vi "Follower16_Final.vi"() -> ()   [LabVIEW 2016]
uses:
  <vilib>/NXT/Block Support/NXT_InputPort.ctl
  <vilib>/NXT/Block Support/NXT_TimerIndex.ctl
  <vilib>/NXT/Block Support/NXT_OutputPort.ctl
  <vilib>/NXT/Dual Mode Library/Sensors/EV3_Gyro_Reset.vi
  <vilib>/NXT/Dual Mode Library/Sensors/EV3_Gyro_Angle.vi
  <vilib>/NXT/Dual Mode Library/Sensors/EV3_Gyro_Rate.vi
  <vilib>/NXT/Dual Mode Library/Sensors/Reset_Timer.vi
  <vilib>/NXT/Dual Mode Library/Sensors/EV3_Color_Reflect.vi
  <vilib>/NXT/Dual Mode Library/Sensors/Read_Timer.vi
  <vilib>/NXT/Dual Mode Library/Sensors/EV3_Ultrasonic_CM.vi
  <vilib>/NXT/Dual Mode Library/Display/drawText_Right.vi
  <vilib>/NXT/Dual Mode Library/prims/inRangeAndCoerce/inRangeAndCoerce_float.vi
  <vilib>/NXT/NXTIO Xnodes/NXTIONodeSubVIs/NXTMoveMotors.vi
  <vilib>/NXT/Dual Mode Library/Display/drawNumber.vi
  <vilib>/NXT/Dual Mode Library/Display/drawNumber_float.vi
  <vilib>/NXT/Dual Mode Library/Motors/Rotation.vi
  <vilib>/NXT/Dual Mode Library/Motors/ResetMotor.vi
  <vilib>/NXT/Dual Mode Library/Sensors/Touch_Pressed.vi
  <vilib>/NXT/Dual Mode Library/Sound/PlayC.vi
  <vilib>/NXT/Dual Mode Library/Display/drawText.vi
  <vilib>/NXT/NXTIO Xnodes/NXTIONodeSubVIs/NXTStopMotors.vi
  <vilib>/NXT/Subs/LVHSConnector.ctl
  <vilib>/NXT/NXTIO Xnodes/AddressXNode/NXTIOAddress.xnode
  <vilib>/NXT/NXTIO Xnodes/NXTIOXNode/NXTIO.xnode
  <vilib>/NXT/LegoClasses/BrickReference/BrickReference.lvclass
panel:
  out "Value (msec)":u32
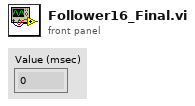
[diagram p1: front panel]
types:
  T1 = typedef "NXT_InputPort.ctl" = u32
  T2 = typedef "LVHSConnector.ctl" = refnum<class "BrickReference.lvclass">
  T3 = typedef "NXT_TimerIndex.ctl" = u8
  T4 = typedef "NXT_OutputPort.ctl" = u8
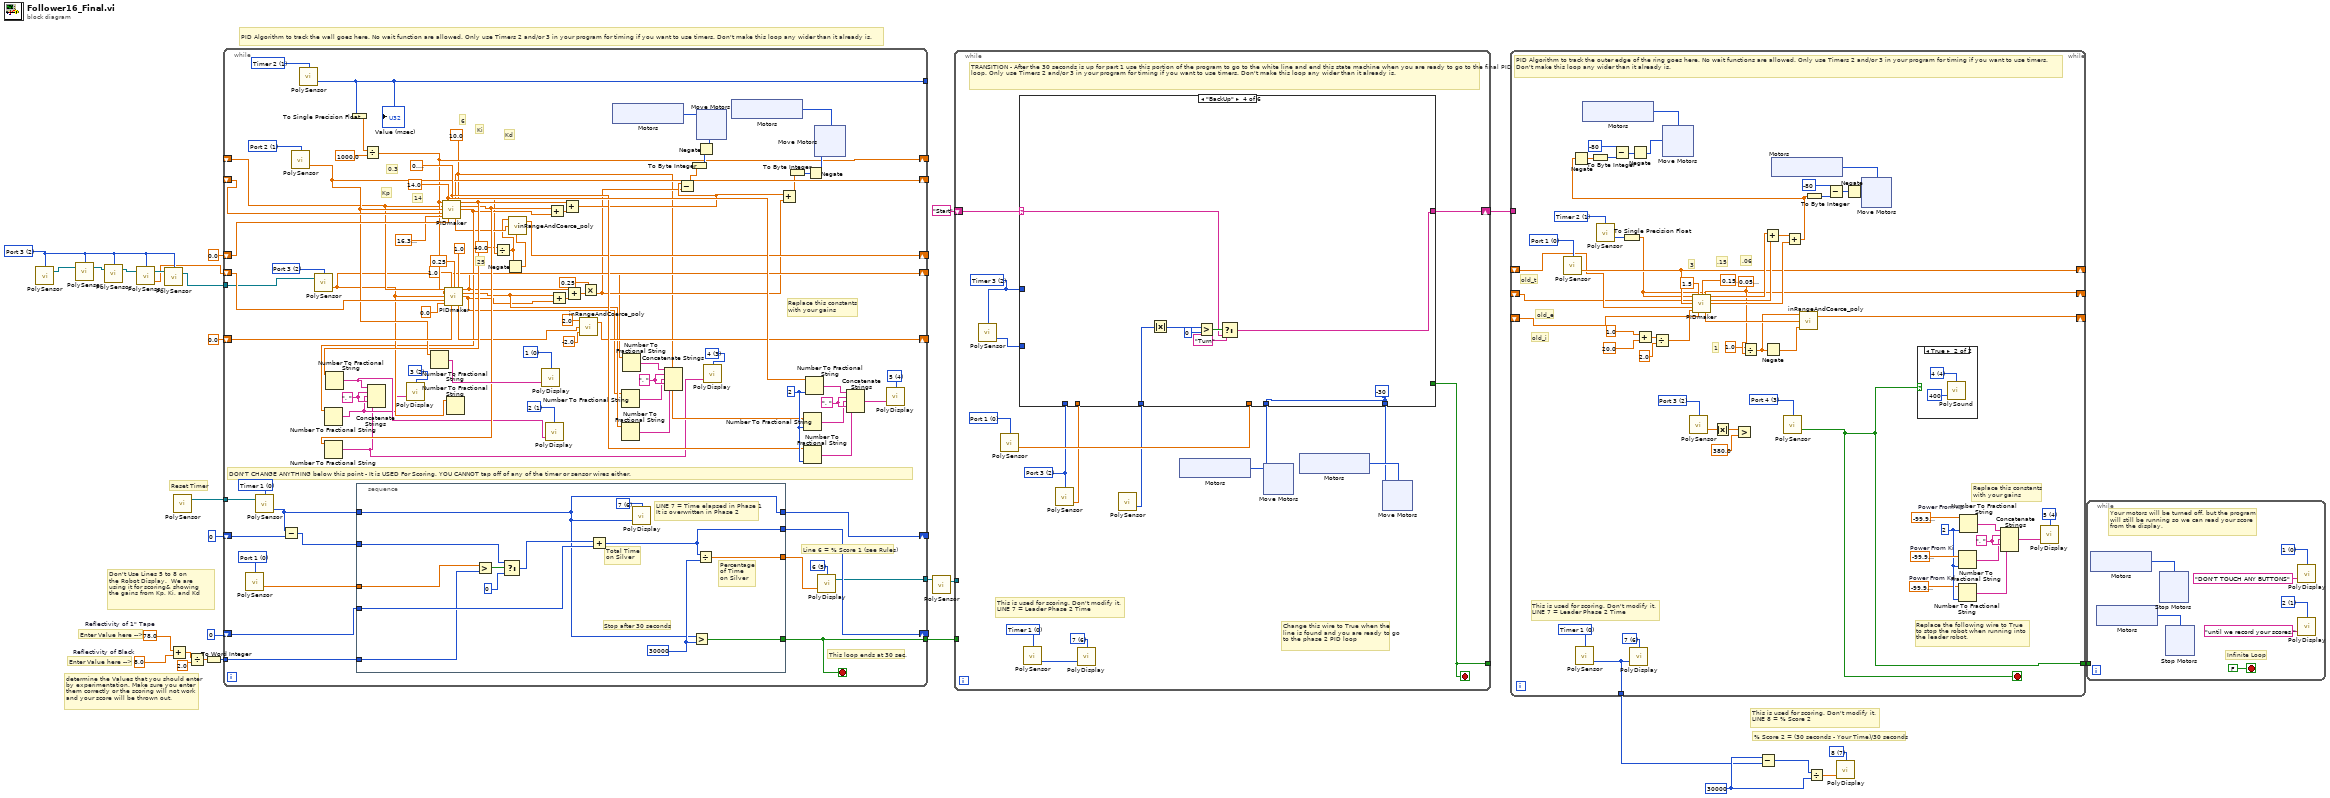
[diagram p0: block diagram]
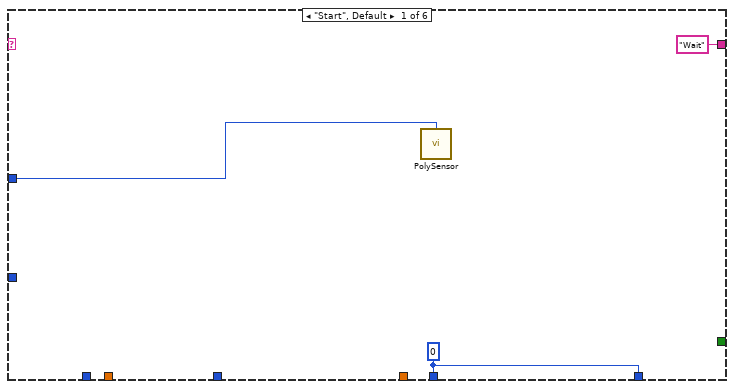
[diagram p3: hidden frame]
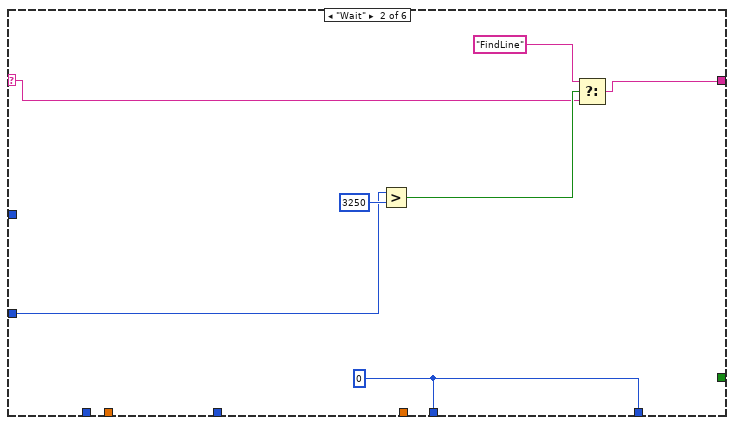
[diagram p4: hidden frame]
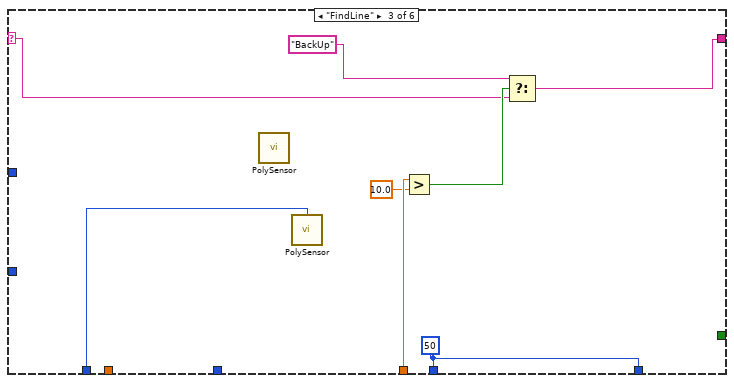
[diagram p5: hidden frame]
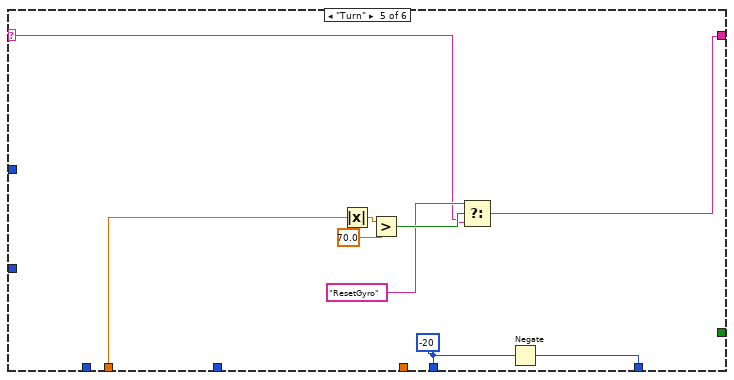
[diagram p6: hidden frame]
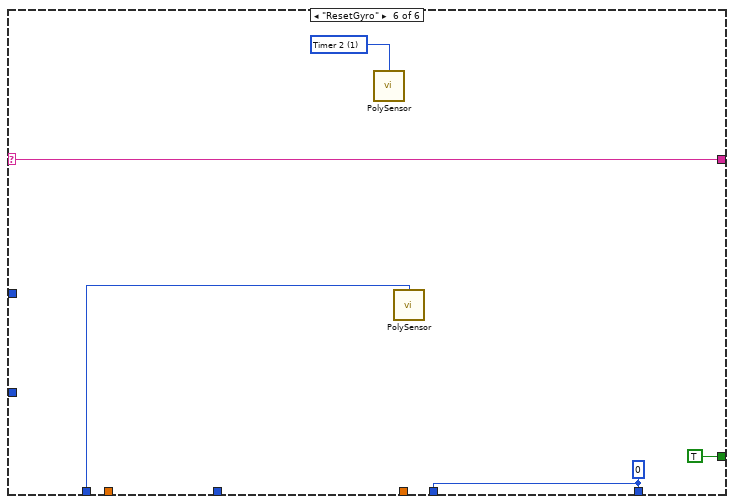
[diagram p7: hidden frame]
diagram:
  w5 = T1 2 items=["Port 1", "Port 2", "Port 3", "Port 4"] ("Port (Port 1)")
  w13 = u32 30000 ("Value (msec)")
  w14 = i16 7 items=["1", "2", "3", "4", "5", "6", "7", "8", "9", "10", "11", "12"] ("Line")
  w20 = 8.0  # Reflectivity of Black
  w19 = 78.0  # Reflectivity of 1" Tape
  # "PID Algorithm to track the wall goes here. No wait function are allowed. Only use Timers 2 and/or 3 in your program for timing if you want to use timers. Don't make this loop any wider than it already is."
  # "This is used for scoring. Don't modify it.\nLINE 8 = % Score 2"
  # "Don't Use Lines 5 to 8 on\nthe Robot Display.  We are \nusing it for scoring& showing \nthe gains from Kp, Ki, and Kd"
  # "% Score 2 = (30 seconds - Your Time)/30 seconds"
  # "Enter Value here -->"
  # "determine the Values that you should enter\nby experimentation. Make sure you enter \nthem correctly or the scoring will not work\nand your score will be thrown out."
  # "Enter Value here -->"
  # "Reset Timer"
  n1 = call-poly <vilib>:"PolySensor.vi"("Port (Port 1)"=w5) -> ("NXT/EV3"=w6:T2)  [unwired: 3 in]
  n2 = call-poly <vilib>:"PolySensor.vi"("NXT/EV3"=w6, "Port (Port 1)"=w5) -> ("NXT/EV3"=w7:T2)  [unwired: 1 in, 1 out]
  n3 = call-poly <vilib>:"PolySensor.vi"("NXT/EV3"=w7, "Port (Port 1)"=w5) -> ("NXT/EV3"=w9:T2)  [unwired: 1 in, 1 out]
  n4 = call-poly <vilib>:"PolySensor.vi"("NXT/EV3"=w9, "Port (Port 1)"=w5) -> ("Degrees"=w1:sgl, "NXT/EV3"=w8:T2)  [unwired: 1 in]
  n5 = call-poly <vilib>:"PolySensor.vi"("NXT/EV3"=w8, "Port (Port 1)"=w5) -> ("NXT/EV3"=w4:T2)  [unwired: 2 in]
  n6 = Add(x=w19, y=w20) -> (x+y=w18:dbl)
  n7 = call-poly <vilib>:"PolySensor.vi"() -> ("NXT/EV3"=w27:T2)  [unwired: 4 in]
  n8 = Divide(x=w18, y=2.0) -> (x/y=w17:dbl)
  n9 = To Word Integer(number=w17) -> (16bit integer=w24:i16)
  n10 = while {
    shift-right: [w112] -> _
    shift-left: i16 0 -> [w116]
    shift-right: [w113] -> _
    shift-left: i16 0 ("Value (msec)") -> [w115]
    tunnel: w27 -> [w111]
    tunnel: [w114] -> w26
    tunnel: w24 -> [w106]
    tunnel: [w102] -> w22
    shift-right: [w47] -> _
    shift-left: sgl 0.0 ("coerced(x)") -> [w83]
    shift-right: [w62] -> _
    shift-left: sgl 0.0 ("coerced(x)") -> [w88]
    shift-right: [w51] -> _
    shift-left: w1 -> [w86]
    tunnel: [w82] -> _
    shift-right: [w57] -> _
    shift-left: _ -> [w56]
    shift-right: [w70] -> _
    shift-left: _ -> [w78]
    tunnel: w4 -> [w50]
    stop <- w114 stop-if-true
    w43 = ", " ("string")
    w40 = i16 3 items=["1", "2", "3", "4", "5", "6", "7", "8", "9", "10", "11", "12"] ("Line")
    w52 = i16 1 items=["1", "2", "3", "4", "5", "6", "7", "8", "9", "10", "11", "12"] ("Line")
    w69 = ", " ("string")
    w68 = i16 2 items=["1", "2", "3", "4", "5", "6", "7", "8", "9", "10", "11", "12"] ("Line")
    w72 = i16 0 items=["1", "2", "3", "4", "5", "6", "7", "8", "9", "10", "11", "12"] ("Line")
    w36 = sgl 10.0 ("Ki")
    w75 = sgl 0.3 ("Kd")
    w76 = sgl 14.0 ("Kp")
    w79 = T1 1 items=["Port 1", "Port 2", "Port 3", "Port 4"] ("Port (Port 1)")
    w84 = T3 1 items=["Timer 1", "Timer 2", "Timer 3"] ("Timer (Timer 1)")
    w87 = T1 2 items=["Port 1", "Port 2", "Port 3", "Port 4"] ("Port (Port 1)")
    w98 = ", " ("string")
    w100 = i16 2 ("precision (6)")
    w101 = i16 4 items=["1", "2", "3", "4", "5", "6", "7", "8", "9", "10", "11", "12"] ("Line")
    w104 = i16 5 items=["1", "2", "3", "4", "5", "6", "7", "8", "9", "10", "11", "12"] ("Line")
    w108 = T1 0 items=["Port 1", "Port 2", "Port 3", "Port 4"] ("Port (Port 3)")
    w109 = T3 0 items=["Timer 1", "Timer 2", "Timer 3"] ("Timer (Timer 1)")
    # "14"
    # "25"
    # "6"
    # "0.3"
    # "Kp"
    # "Kd"
    # "Ki"
    # "Replace this constants\nwith your gains"
    # "DON'T CHANGE ANYTHING below this point - It is USED For Scoring. YOU CANNOT tap off of any of the timer or sensor wires either."
    # "Line 6 = % Score 1 (see Rules)"
    # "This loop ends at 30 sec."
    n11 = call-poly <vilib>:"PolySensor.vi"("Port (Port 1)"=w108) -> ("Scaled Value"=w107:sgl)  [unwired: 2 in, 1 out]
    n12 = call-poly <vilib>:"PolySensor.vi"("NXT/EV3"=w111, "Timer (Timer 1)"=w109) -> ("Value (msec)"=w110:u32)  [unwired: 1 in, 1 out]
    n13 = Subtract(x=w110, y=w115) -> (x-y=w105:u32)
    n14 = call-poly <vilib>:"PolySensor.vi"("Port (Port 1)"=w79) -> ("Centimeters"=w70:sgl)  [unwired: 2 in, 1 out]
    n15 = call-poly <vilib>:"PolySensor.vi"("Timer (Timer 1)"=w84) -> ("Value (msec)"=w82:u32)  [unwired: 2 in, 1 out]
    "Value (msec)" <- w82
    n16 = call-poly <vilib>:"PolySensor.vi"("NXT/EV3"=w50, "Port (Port 1)"=w87) -> ("Degrees"=w51:sgl)  [unwired: 1 in, 1 out]
    n17 = To Single Precision Float(number=w82) -> (single precision float=w80:sgl)
    n18 = stacked-sequence {
      tunnel: w116 -> [w145]
      tunnel: [w135] -> w103
      tunnel: w110 -> [w133]
      tunnel: [w144] -> w114
      tunnel: w107 -> [w139]
      tunnel: w105 -> [w141]
      tunnel: [w133] -> w113
      tunnel: [w137] -> w112
      tunnel: w106 -> [w138]
      frame #0 {
        w134 = i16 6 items=["1", "2", "3", "4", "5", "6", "7", "8", "9", "10", "11", "12"] ("Line")
        w136 = u32 30000 ("Value (msec)")
        # "LINE 7 = Time elapsed in Phase 1\nIt is overwritten in Phase 2"
        # "Percentage\nof Time\non Silver"
        # "Stop after 30 seconds"
        # "Total Time\non Silver"
        n19 = Greater?(x=w139, y=w138) -> (0:w142:bool)
        n20 = Select(t=w141, s=w142, f=i16 0) -> (s? t:f=w140:u32)
        n21 = Add(x=w140, y=w145) -> (x+y=w137:u32)
        n22 = call-poly <vilib>:"PolyDisplay.vi"("number"=w133, "Line"=w134) -> ()  [unwired: 2 in, 1 out]
        n23 = Greater?(x=w133, y=w136) -> (0:w144:bool)
        n24 = Divide(x=w137, y=w136) -> (x/y=w135:dbl)
      }
    }
    n25 = Divide(x=w80, y=sgl 1000.0) -> (x/y=w57:sgl)
    n26 = Number To Fractional String(number=w70) -> (F-format string=w71:string)  [unwired: 3 in]
    n27 = call "PIDmaker.vi"("New Time"=w57, "Kp"=w76, "Kd"=w75, "Ki"=w36, "Old Time"=w56, "New Value"=w70, "Old Value"=w78, "Desired Value"=sgl 16.4, "Integral In"=w83) -> ("P out"=w67:sgl, "D out"=w66:sgl, "I out"=w49:sgl, "Integral Out"=w48:sgl)  [unwired: 3 in]
    n28 = Number To Fractional String(number=w49) -> (F-format string=w31:string)  [unwired: 3 in]
    n29 = Number To Fractional String(number=w66) -> (F-format string=w30:string)  [unwired: 3 in]
    n30 = Number To Fractional String(number=w67) -> (F-format string=w32:string)  [unwired: 3 in]
    n31 = Concatenate Strings(w32, w69, w31, w69, w30) -> ()  [unwired: 1 out]
    n32 = call-poly <vilib>:"PolyDisplay.vi"("Text"=w31, "Line"=w68) -> ()  [unwired: 2 in, 1 out]
    n33 = call "PIDmaker.vi"("New Time"=w57, "Kp"=sgl 1.0, "Kd"=sgl 0.25, "Ki"=sgl 1.0, "Old Time"=w56, "New Value"=w51, "Old Value"=w86, "Desired Value"=sgl 0.0, "Integral In"=w88) -> ("P out"=w39:sgl, "D out"=w38:sgl, "I out"=w37:sgl, "Integral Out"=w63:sgl)  [unwired: 3 in]
    n34 = Number To Fractional String(number=w51) -> ()  [unwired: 3 in, 1 out]
    n35 = Divide(x=sgl 40.0, y=w36) -> (x/y=w34:sgl)
    n36 = Negate(x=w34) -> (-x=w33:sgl)
    n37 = call-poly <vilib>:"inRangeAndCoerce_poly.vi"("lower limit"=w33, "x"=w48, "upper limit"=w34) -> ("coerced(x)"=w47:sgl)  [unwired: 1 out]
    n38 = call-poly <vilib>:"PolyDisplay.vi"("Text"=w71, "Line"=w72) -> ()  [unwired: 2 in, 1 out]
    n39 = call-poly <vilib>:"PolyDisplay.vi"("Text"=w32, "Line"=w52) -> ()  [unwired: 2 in, 1 out]
    n40 = Add(x=w66, y=w49) -> (x+y=w92:sgl)
    n41 = Add(x=w38, y=w37) -> (x+y=w89:sgl)
    n42 = Add(x=w67, y=w92) -> (x+y=w60:sgl)
    n43 = Add(x=w39, y=w89) -> (x+y=w58:sgl)
    n44 = call-poly <vilib>:"inRangeAndCoerce_poly.vi"("lower limit"=sgl -2.0, "x"=w63, "upper limit"=sgl 2.0) -> ("coerced(x)"=w62:sgl)  [unwired: 1 out]
    n45 = Multiply(x=sgl 0.25, y=w58) -> (x*y=w46:sgl)
    n46 = xnode "Motors"() -> ("Motor"=w94:T4)
    n47 = Number To Fractional String(number=w37) -> (F-format string=w42:string)  [unwired: 3 in]
    n48 = Number To Fractional String(number=w38) -> (F-format string=w41:string)  [unwired: 3 in]
    n49 = Number To Fractional String(number=w39) -> (F-format string=w44:string)  [unwired: 3 in]
    n50 = Concatenate Strings(w44, w43, w42, w43, w41) -> ()  [unwired: 1 out]
    n51 = Subtract(x=w60, y=w46) -> (x-y=w61:sgl)
    n52 = To Byte Integer(number=w61) -> (8bit integer=w73:i8)
    n53 = Negate(x=w73) -> (-x=w65:i8)
    n54 = xnode "Move Motors"("Power/Speed 1"=w65, "Motors"=w94) -> ()  [unwired: 1 in, 1 out]
    n55 = call-poly <vilib>:"PolyDisplay.vi"("Text"=w30, "Line"=w40) -> ()  [unwired: 2 in, 1 out]
    n56 = xnode "Motors"() -> ("Motor"=w93:T4)
    n57 = Add(x=w60, y=w46) -> (x+y=w59:sgl)
    n58 = To Byte Integer(number=w59) -> (8bit integer=w74:i8)
    n59 = Number To Fractional String(number=w36, precision (6)=w100) -> (F-format string=w97:string)  [unwired: 2 in]
    n60 = Number To Fractional String(number=w75, precision (6)=w100) -> (F-format string=w96:string)  [unwired: 2 in]
    n61 = Number To Fractional String(number=w76, precision (6)=w100) -> (F-format string=w99:string)  [unwired: 2 in]
    n62 = Negate(x=w74) -> (-x=w64:i8)
    n63 = xnode "Move Motors"("Power/Speed 1"=w64, "Motors"=w93) -> ()  [unwired: 1 in, 1 out]
    n64 = call-poly <vilib>:"PolyDisplay.vi"("number"=w103, "Line"=w104) -> ("NXT/EV3"=w102:T2)  [unwired: 2 in]
    n65 = Concatenate Strings(w99, w98, w97, w98, w96) -> (w95:string)
    n66 = call-poly <vilib>:"PolyDisplay.vi"("Text"=w95, "Line"=w101) -> ()  [unwired: 2 in, 1 out]
  }
  n67 = call-poly <vilib>:"PolySensor.vi"("NXT/EV3"=w22) -> ("NXT/EV3"=w21:T2)  [unwired: 3 in]
  n68 = while {
    tunnel: w26 -> [_]
    shift-right: [w148] -> w15
    shift-left: "Start" -> [w147]
    tunnel: w21 -> [_]
    tunnel: [w146] -> _
    stop <- w146 stop-if-true
    w151 = T1 2 items=["Port 1", "Port 2", "Port 3", "Port 4"] ("Port (Port 1)")
    w153 = T1 0 items=["Port 1", "Port 2", "Port 3", "Port 4"] ("Port (Port 1)")
    w157 = T3 2 items=["Timer 1", "Timer 2", "Timer 3"] ("Timer (Timer 1)")
    w160 = i16 6 items=["1", "2", "3", "4", "5", "6", "7", "8", "9", "10", "11", "12"] ("Line")
    w162 = T3 0 items=["Timer 1", "Timer 2", "Timer 3"] ("Timer (Timer 1)")
    # "This is used for scoring. Don't modify it.\nLINE 7 = Leader Phase 2 Time"
    # "Change this wire to True when the line is found and you are ready to go to the phase 2 PID loop"
    # "TRANSITION - After the 30 seconds is up for part 1 use this portion of the program to go to the white line and end this state machine when you are ready to go to the final PID control loop. Only use Timers 2 and/or 3 in your program for timing if you want to use timers. Don't make this loop any wider than it already is."
    n69 = call-poly <vilib>:"PolySensor.vi"("Timer (Timer 1)"=w157) -> ("Value (msec)"=w156:u32)  [unwired: 2 in, 1 out]
    n70 = call-poly <vilib>:"PolySensor.vi"("Port (Port 1)"=w153) -> ("Scaled Value"=w152:sgl)  [unwired: 2 in, 1 out]
    n71 = call-poly <vilib>:"PolySensor.vi"("Timer (Timer 1)"=w162) -> ("Value (msec)"=w161:u32)  [unwired: 2 in, 1 out]
    n72 = call-poly <vilib>:"PolySensor.vi"("Port (Port 1)"=w151) -> ("Degrees"=w150:sgl)  [unwired: 2 in, 1 out]
    n73 = call-poly <vilib>:"PolyDisplay.vi"("number"=w161, "Line"=w160) -> ()  [unwired: 2 in, 1 out]
    n74 = call-poly <vilib>:"PolySensor.vi"() -> ("Angle of Rotation"=w149:i32)  [unwired: 3 in, 1 out]
    n75 = case shown="\"BackUp\"" w147 {
      selector: w147 -> [_ w184 w191 w199 w206 w216]
      tunnel: ["Wait" w187 w193 w197 w205 w216] -> w148
      tunnel: w157 -> [w181 _ _ _ _ _]
      tunnel: w156 -> [_ w183 _ _ _ _]
      tunnel: [w179 w182 w189 w204 w213 w215] -> w155
      tunnel: [w179 w182 w189 w204 w212 w215] -> w154
      tunnel: w152 -> [_ _ w196 _ _ _]
      tunnel: w151 -> [_ _ w190 _ _ w218]
      tunnel: w150 -> [_ _ _ _ w211 _]
      tunnel: w149 -> [_ _ _ w203 _ _]
      tunnel: [_ _ _ _ _ TRUE] -> w146
      frame "Start", Default {
        w179 = 0
        n76 = call-poly <vilib>:"PolySensor.vi"("Timer (Timer 1)"=w181) -> ()  [unwired: 3 in, 1 out]
      }
      frame "Wait" {
        w182 = 0
        n77 = Greater?(x=w183, y=u32 3250) -> (0:w185:bool)
        n78 = Select(t="FindLine", s=w185, f=w184) -> (s? t:f=w187:string)
      }
      frame "FindLine" {
        w189 = 50
        n79 = call-poly <vilib>:"PolySensor.vi"() -> ()  [unwired: 4 in, 1 out]
        n80 = call-poly <vilib>:"PolySensor.vi"("Port (Port 1)"=w190) -> ()  [unwired: 3 in, 1 out]
        n81 = Greater?(x=w196, y=sgl 10.0) -> (0:w194:bool)
        n82 = Select(t="BackUp", s=w194, f=w191) -> (s? t:f=w193:string)
      }
      frame "BackUp" {
        w204 = -30
        n83 = Absolute Value(x=w203) -> (abs(x)=w201:i32)
        n84 = Greater?(x=w201, y=0) -> (0:w200:bool)
        n85 = Select(t="Turn", s=w200, f=w199) -> (s? t:f=w197:string)
      }
      frame "Turn" {
        w213 = -20
        n86 = Absolute Value(x=w211) -> (abs(x)=w210:sgl)
        n87 = Greater?(x=w210, y=sgl 70.0) -> (0:w208:bool)
        n88 = Select(t="ResetGyro", s=w208, f=w206) -> (s? t:f=w205:string)
        n89 = Negate(x=w213) -> (-x=w212:i32)
      }
      frame "ResetGyro" {
        w214 = T3 1 items=["Timer 1", "Timer 2", "Timer 3"] ("Timer (Timer 1)")
        w215 = 0
        n90 = call-poly <vilib>:"PolySensor.vi"("Timer (Timer 1)"=w214) -> ()  [unwired: 3 in, 1 out]
        n91 = call-poly <vilib>:"PolySensor.vi"("Port (Port 1)"=w218) -> ()  [unwired: 3 in, 1 out]
      }
    }
    n92 = xnode "Motors"() -> ("Motor"=w159:T4)
    n93 = xnode "Move Motors"("Power/Speed 1"=w155, "Motors"=w159) -> ()  [unwired: 1 in, 1 out]
    n94 = xnode "Motors"() -> ("Motor"=w158:T4)
    n95 = xnode "Move Motors"("Power/Speed 1"=w154, "Motors"=w158) -> ()  [unwired: 1 in, 1 out]
  }
  n96 = while {
    tunnel: [w226] -> w16
    tunnel: w15 -> [_]
    tunnel: [w272] -> w12
    shift-right: [w233] -> _
    shift-left: _ -> [w229]
    shift-right: [w232] -> _
    shift-left: _ -> [w228]
    shift-right: [w231] -> _
    shift-left: _ -> [w230]
    stop <- w226 stop-if-true
    w227 = T1 3 items=["Port 1", "Port 2", "Port 3", "Port 4"] ("Port (Port 1)")
    w237 = T1 2 items=["Port 1", "Port 2", "Port 3", "Port 4"] ("Port (Port 1)")
    w245 = sgl 0.05 ("Ki")
    w259 = T3 1 items=["Timer 1", "Timer 2", "Timer 3"] ("Timer (Timer 1)")
    w260 = T1 0 items=["Port 1", "Port 2", "Port 3", "Port 4"] ("Port (Port 1)")
    w265 = ", " ("string")
    w268 = i16 2 ("precision (6)")
    w267 = sgl -99.9  # Power From Kd
    w269 = sgl -99.9  # Power From Ki
    w270 = sgl -99.9  # Power From Kp
    w271 = i16 4 items=["1", "2", "3", "4", "5", "6", "7", "8", "9", "10", "11", "12"] ("Line")
    w273 = i16 6 items=["1", "2", "3", "4", "5", "6", "7", "8", "9", "10", "11", "12"] ("Line")
    w274 = T3 0 items=["Timer 1", "Timer 2", "Timer 3"] ("Timer (Timer 1)")
    # "3"
    # ".15"
    # ".06"
    # "1"
    # "old_i"
    # "old_e"
    # "old_t"
    # "Replace this constants\nwith your gains"
    # "This is used for scoring. Don't modify it.\nLINE 7 = Leader Phase 2 Time"
    # "PID Algorithm to track the outer edge of the ring goes here. No wait functions are allowed. Only use Timers 2 and/or 3 in your program for timing if you want to use timers.\nDon't make this loop any wider than it already is."
    # "Replace the following wire to True\nto stop the robot when running into \nthe leader robot."
    n97 = call-poly <vilib>:"PolySensor.vi"("Port (Port 1)"=w260) -> ("Scaled Value"=w233:sgl)  [unwired: 2 in, 1 out]
    n98 = call-poly <vilib>:"PolySensor.vi"("Timer (Timer 1)"=w274) -> ("Value (msec)"=w272:u32)  [unwired: 2 in, 1 out]
    n99 = xnode "Motors"() -> ("Motor"=w242:T4)
    n100 = call-poly <vilib>:"PolySensor.vi"("Timer (Timer 1)"=w259) -> ("Value (msec)"=w258:u32)  [unwired: 2 in, 1 out]
    n101 = To Single Precision Float(number=w258) -> (single precision float=w232:sgl)
    n102 = call-poly <vilib>:"PolyDisplay.vi"("number"=w272, "Line"=w273) -> ()  [unwired: 2 in, 1 out]
    n103 = Add(x=sgl 1.0, y=sgl 20.0) -> (x+y=w255:sgl)
    n104 = Divide(x=w255, y=sgl 2.0) -> (x/y=w252:sgl)
    n105 = call-poly <vilib>:"PolySensor.vi"("Port (Port 1)"=w237) -> ("Degrees"=w236:sgl)  [unwired: 2 in, 1 out]
    n106 = call "PIDmaker.vi"("New Time"=w232, "Kp"=sgl 1.5, "Kd"=sgl 0.15, "Ki"=w245, "Old Time"=w228, "New Value"=w233, "Old Value"=w229, "Desired Value"=w252, "Integral In"=w230) -> ("P out"=w248:sgl, "D out"=w247:sgl, "I out"=w246:sgl, "Integral Out"=w251:sgl)  [unwired: 3 in]
    n107 = Absolute Value(x=w236) -> (abs(x)=w234:sgl)
    n108 = Greater?(x=w234, y=sgl 380.0) -> ()  [unwired: 1 out]
    n109 = Divide(x=sgl 1.0, y=w245) -> (x/y=w243:sgl)
    n110 = Add(x=w248, y=w247) -> (x+y=w249:sgl)
    n111 = Negate(x=w243) -> (-x=w244:sgl)
    n112 = xnode "Motors"() -> ("Motor"=w261:T4)
    n113 = call-poly <vilib>:"PolySensor.vi"("Port (Port 1)"=w227) -> ("Yes / No"=w226:bool)  [unwired: 2 in, 1 out]
    n114 = Add(x=w249, y=w246) -> (x+y=w220:sgl)
    n115 = Negate(x=w220) -> (-x=w221:sgl)
    n116 = To Byte Integer(number=w221) -> (8bit integer=w225:i8)
    n117 = Subtract(x=i8 -80, y=w225) -> (x-y=w223:i8)
    n118 = Negate(x=w223) -> (-x=w222:i8)
    n119 = xnode "Move Motors"("Power/Speed 1"=w222, "Motors"=w242) -> ()  [unwired: 1 in, 1 out]
    n120 = call-poly <vilib>:"inRangeAndCoerce_poly.vi"("lower limit"=w244, "x"=w251, "upper limit"=w243) -> ("coerced(x)"=w231:sgl)  [unwired: 1 out]
    n121 = To Byte Integer(number=w220) -> (8bit integer=w241:i8)
    n122 = Subtract(x=i8 -80, y=w241) -> (x-y=w239:i8)
    n123 = Negate(x=w239) -> (-x=w238:i8)
    n124 = xnode "Move Motors"("Power/Speed 1"=w238, "Motors"=w261) -> ()  [unwired: 1 in, 1 out]
    n125 = case shown="True" w226 {
      frame False {
      }
      frame True {
        w275 = u16 4 items=["3"=3, "4"=4, "5"=5, "6"=6, "7"=7] ("Octave")
        n126 = call-poly <vilib>:"PolySound.vi"("Duration (500 ms)"=u16 400, "Octave"=w275) -> ()  [unwired: 2 in, 1 out]
      }
    }
    n127 = Number To Fractional String(number=w269, precision (6)=w268) -> (F-format string=w264:string)  [unwired: 2 in]
    n128 = Number To Fractional String(number=w267, precision (6)=w268) -> (F-format string=w263:string)  [unwired: 2 in]
    n129 = Number To Fractional String(number=w270, precision (6)=w268) -> (F-format string=w266:string)  [unwired: 2 in]
    n130 = Concatenate Strings(w266, w265, w264, w265, w263) -> (w262:string)
    n131 = call-poly <vilib>:"PolyDisplay.vi"("Text"=w262, "Line"=w271) -> ()  [unwired: 2 in, 1 out]
  }
  n132 = Subtract(x=w13, y=w12) -> (x-y=w11:u32)
  n133 = Divide(x=w11, y=w13) -> (x/y=w10:dbl)
  n134 = call-poly <vilib>:"PolyDisplay.vi"("number"=w10, "Line"=w14) -> ()  [unwired: 2 in, 1 out]
  n135 = while {
    tunnel: w16 -> [_]
    stop <- FALSE stop-if-true
    w293 = i16 1 items=["1", "2", "3", "4", "5", "6", "7", "8", "9", "10", "11", "12"] ("Line")
    w296 = i16 0 items=["1", "2", "3", "4", "5", "6", "7", "8", "9", "10", "11", "12"] ("Line")
    # "Your motors will be turned off, but the program\nwill still be running so we can read your score\nfrom the display."
    # "Infinite Loop"
    n136 = xnode "Motors"() -> ("Motor"=w298:T4)
    n137 = xnode "Motors"() -> ("Motor"=w297:T4)
    n138 = xnode "Stop Motors"("Motors"=w298) -> ()  [unwired: 1 in, 1 out]
    n139 = xnode "Stop Motors"("Motors"=w297) -> ()  [unwired: 1 in, 1 out]
    n140 = call-poly <vilib>:"PolyDisplay.vi"("Text"="DON'T TOUCH ANY BUTTONS", "Line"=w296) -> ()  [unwired: 2 in, 1 out]
    n141 = call-poly <vilib>:"PolyDisplay.vi"("Text"="until we record your scores.", "Line"=w293) -> ()  [unwired: 2 in, 1 out]
  }
